vi "Main.vi"() -> ()   [LabVIEW 2015]
uses:
  <userlib>/LV Exceptions v1/LV Exceptions v1.lvlib
panel:
  in  "Calculate":bool
  in  "Expression":string
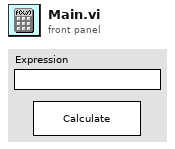
[diagram p1: front panel]
types:
  T1 = typedef "Operand.ctl" = enum16{"/", "@"}
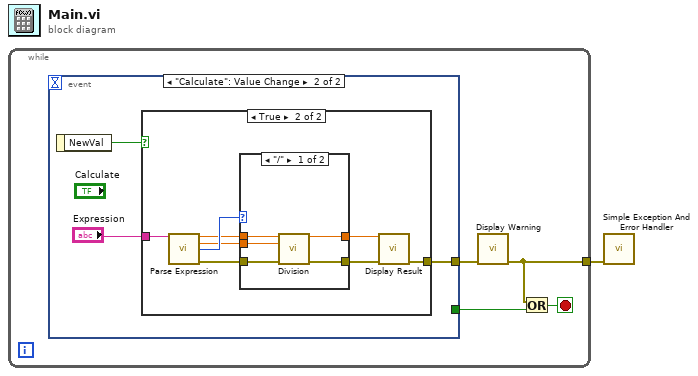
[diagram p0: block diagram]
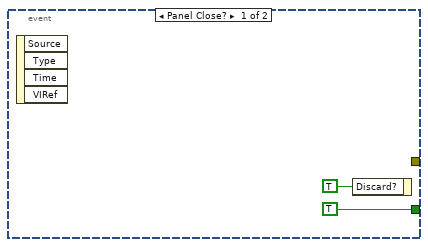
[diagram p2: hidden frame]
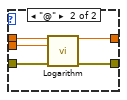
[diagram p4: hidden frame]
diagram:
  n1 = while {
    tunnel: [w2] -> w1
    stop <- w4 stop-if-true
    n2 = event shown="[1] \"Calculate\": Value Change" {
      selector: _ -> [_ _]
      dyn-events: _ -> [_ _]
      timeout: _ -> [_ _]
      tunnel: [TRUE ("Discard?") _] -> w5
      tunnel: [_ w8] -> w3
      event Panel Close? {
        n3 = event-data() -> ()  [unwired: 1 in, 4 out]
        n4 = event-data("Discard?"=TRUE) -> ()  [unwired: 1 in, 1 out]
      }
      event "Calculate": Value Change {
        n5 = event-data() -> ("NewVal"=w10:bool)  [unwired: 1 in]
        n6 = case shown="True" w10 {
          tunnel: "Expression" -> [_ w18]
          tunnel: [_ w11] -> w8
          frame False {
          }
          frame True {
            n7 = call "Parse Expression.vi"("expression"=w18) -> ("x"=w16:dbl, "y"=w15:dbl, "operand"=w17:T1, "error out"=w14:errorcluster)  [unwired: 11 in]
            n8 = case shown="\"/\"" w17 {
              tunnel: w16 -> [w23 w28]
              tunnel: w15 -> [w22 w27]
              tunnel: w14 -> [w21 w26]
              tunnel: [w20 w25] -> w13
              tunnel: [w19 w24] -> w12
              frame "/" {
                n9 = call "Division.vi"("x"=w23, "y"=w22, "error in (no error)"=w21) -> ("quotient"=w20:dbl, "error out"=w19:errorcluster)  [unwired: 11 in]
              }
              frame "@" {
                n10 = call "Logarithm.vi"("argument"=w28, "base"=w27, "error in (no error)"=w26) -> ("exponent"=w25:dbl, "error out"=w24:errorcluster)  [unwired: 11 in]
              }
            }
            n11 = call "Display Result.vi"("exponent"=w13, "error in (no error)"=w12) -> ("error out"=w11:errorcluster)  [unwired: 13 in]
          }
        }
      }
    }
    n12 = call "Display Warning.vi"("error in (no error)"=w3) -> ("error out"=w2:errorcluster)  [unwired: 14 in]
    n13 = Or(x=w2, y=w5) -> (x .or. y?=w4:bool)
  }
  n14 = call <userlib>:"Simple Exception And Error Handler.vi"("error in (no error)"=w1) -> ()  [unwired: 14 in, 1 out]
